vi "MCS_VGap_GapChange.vi"(0 "System Index In":u32, 1 "Gap Change (um)":i32, 2 "Step Change (um)":i32, 3 "error in (no error)":errorcluster, 4 "Stage Delay (ms)":i32) -> (5 "error out":errorcluster)   [LabVIEW 2010]
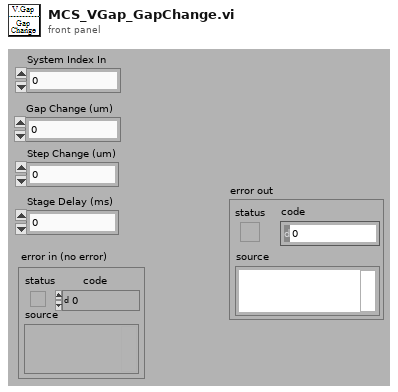
[diagram p1: front panel]
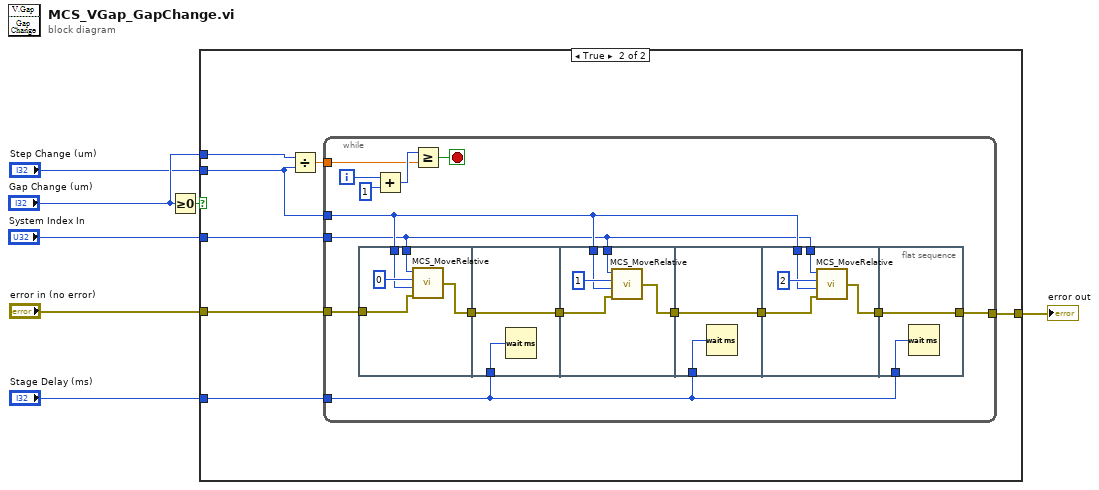
[diagram p0: block diagram]
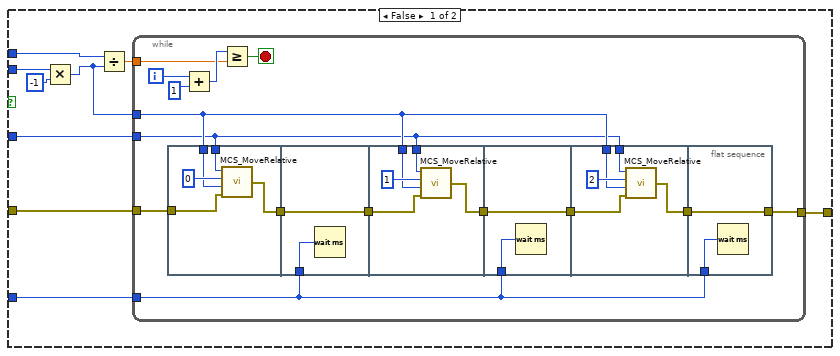
[diagram p2: hidden frame]
diagram:
  n1 = Greater Or Equal To 0?(x="Gap Change (um)") -> (x >= 0?=w7:bool)
  n2 = case shown="True" w7 {
    tunnel: "Gap Change (um)" -> [w12 w59]
    tunnel: "Step Change (um)" -> [w15 w56]
    tunnel: "System Index In" -> [w11 w57]
    tunnel: "error in (no error)" -> [w10 w55]
    tunnel: "Stage Delay (ms)" -> [w9 w54]
    tunnel: [w8 w53] -> w1
    frame False {
      n3 = Multiply(x=w15, y=-1) -> (x*y=w13:i32)
      n4 = Divide(x=w12, y=w13) -> (x/y=w16:dbl)
      n5 = while {
        tunnel: w16 -> [w28]
        tunnel: w11 -> [w20]
        tunnel: w13 -> [w21]
        tunnel: w10 -> [w26]
        tunnel: w9 -> [w18]
        tunnel: [w17] -> w8
        i -> [w31]
        stop <- w27 stop-if-true
        n6 = flat-sequence {
          tunnel: w20 -> [w35]
          tunnel: w21 -> [w34]
          tunnel: w26 -> [w33]
          tunnel: [w32] -> w25
          tunnel: w25 -> [w38]
          tunnel: w18 -> [w37]
          tunnel: [w38] -> w24
          tunnel: w24 -> [w42]
          tunnel: w21 -> [w41]
          tunnel: w20 -> [w40]
          tunnel: [w39] -> w23
          tunnel: w23 -> [w45]
          tunnel: w18 -> [w44]
          tunnel: [w45] -> w22
          tunnel: w22 -> [w49]
          tunnel: w21 -> [w48]
          tunnel: w20 -> [w47]
          tunnel: [w46] -> w19
          tunnel: [w52] -> w17
          tunnel: w19 -> [w52]
          tunnel: w18 -> [w51]
          frame #0 {
            n7 = call "MCS_MoveRelative.vi"("error in (no error)"=w33, "Moving Distance (um)"=w34, "Channel Index In"=u32 0, "System Index In"=w35) -> ("error out"=w32:errorcluster)
          }
          frame #1 {
            n8 = Wait (ms)(milliseconds to wait=w37) -> ()  [unwired: 1 out]
          }
          frame #2 {
            n9 = call "MCS_MoveRelative.vi"("error in (no error)"=w42, "Moving Distance (um)"=w41, "Channel Index In"=u32 1, "System Index In"=w40) -> ("error out"=w39:errorcluster)
          }
          frame #3 {
            n10 = Wait (ms)(milliseconds to wait=w44) -> ()  [unwired: 1 out]
          }
          frame #4 {
            n11 = call "MCS_MoveRelative.vi"("error in (no error)"=w49, "Moving Distance (um)"=w48, "Channel Index In"=u32 2, "System Index In"=w47) -> ("error out"=w46:errorcluster)
          }
          frame #5 {
            n12 = Wait (ms)(milliseconds to wait=w51) -> ()  [unwired: 1 out]
          }
        }
        n13 = Add(x=w31, y=1) -> (x+y=w29:i32)
        n14 = Greater Or Equal?(x=w29, y=w28) -> (x >= y?=w27:bool)
      }
    }
    frame True {
      n15 = Divide(x=w59, y=w56) -> (x/y=w58:dbl)
      n16 = while {
        tunnel: w58 -> [w71]
        tunnel: w57 -> [w63]
        tunnel: w56 -> [w64]
        tunnel: w55 -> [w69]
        tunnel: w54 -> [w61]
        tunnel: [w60] -> w53
        i -> [w74]
        stop <- w70 stop-if-true
        n17 = flat-sequence {
          tunnel: w63 -> [w78]
          tunnel: w64 -> [w77]
          tunnel: w69 -> [w76]
          tunnel: [w75] -> w68
          tunnel: w68 -> [w81]
          tunnel: w61 -> [w80]
          tunnel: [w81] -> w67
          tunnel: w67 -> [w85]
          tunnel: w64 -> [w84]
          tunnel: w63 -> [w83]
          tunnel: [w82] -> w66
          tunnel: w66 -> [w88]
          tunnel: w61 -> [w87]
          tunnel: [w88] -> w65
          tunnel: w65 -> [w92]
          tunnel: w64 -> [w91]
          tunnel: w63 -> [w90]
          tunnel: [w89] -> w62
          tunnel: [w95] -> w60
          tunnel: w62 -> [w95]
          tunnel: w61 -> [w94]
          frame #0 {
            n18 = call "MCS_MoveRelative.vi"("error in (no error)"=w76, "Moving Distance (um)"=w77, "Channel Index In"=u32 0, "System Index In"=w78) -> ("error out"=w75:errorcluster)
          }
          frame #1 {
            n19 = Wait (ms)(milliseconds to wait=w80) -> ()  [unwired: 1 out]
          }
          frame #2 {
            n20 = call "MCS_MoveRelative.vi"("error in (no error)"=w85, "Moving Distance (um)"=w84, "Channel Index In"=u32 1, "System Index In"=w83) -> ("error out"=w82:errorcluster)
          }
          frame #3 {
            n21 = Wait (ms)(milliseconds to wait=w87) -> ()  [unwired: 1 out]
          }
          frame #4 {
            n22 = call "MCS_MoveRelative.vi"("error in (no error)"=w92, "Moving Distance (um)"=w91, "Channel Index In"=u32 2, "System Index In"=w90) -> ("error out"=w89:errorcluster)
          }
          frame #5 {
            n23 = Wait (ms)(milliseconds to wait=w94) -> ()  [unwired: 1 out]
          }
        }
        n24 = Add(x=w74, y=1) -> (x+y=w72:i32)
        n25 = Greater Or Equal?(x=w72, y=w71) -> (x >= y?=w70:bool)
      }
    }
  }
  "error out" <- w1
